vi "Actor Core.vi"(8 "error in":errorcluster, 11 "Recipe Window in":refnum<class "Recipe Window.lvclass">) -> (0 "error out":errorcluster, 3 "Actor out":refnum<class "Actor.lvclass">)   [LabVIEW 2021, in "Recipe.lvlib" / "Recipe Window.lvclass"]
doc: "The user interface for this panel.\n\n----\nPlease see the following web address for additional documentation and tutorial information:\nhttp://www.mooregoodideas.com/mgi-panel-manager/\n\nAuthor: Derek Trepanier\n\nCopyright (c) 2018, Moore Good Ideas, Inc.\n\nAll rights reserved.\n\nRedistribution and use in source and binary forms, with or without modification, are permitted provided that the following conditions are met:\n\n * Redistributions of source code must retain the above copyright notice, this list of conditions and the following disclaimer.\n * Redistributions in binary form must reproduce the above copyright notice, this list of conditions and the following disclaimer in the documentation and/or other materials provided with the distribution.\n * Neither the name of Moore Good Ideas, Inc. nor the names of its contributors may be used to endorse or promote products derived from this software without specific prior written permission.\n\nTHIS SOFTWARE IS PROVIDED BY THE COPYRIGHT HOLDERS AND CONTRIBUTORS \"AS IS\" AND ANY EXPRESS OR IMPLIED WARRANTIES, INCLUDING, BUT NOT LIMITED TO, THE IMPLIED WARRANTIES OF MERCHANTABILITY AND FITNESS FOR A PARTICULAR PURPOSE ARE DISCLAIMED. IN NO EVENT SHALL THE COPYRIGHT OWNER OR CONTRIBUTORS BE LIABLE FOR ANY DIRECT, INDIRECT, INCIDENTAL, SPECIAL, EXEMPLARY, OR CONSEQUENTIAL DAMAGES (INCLUDING, BUT NOT LIMITED TO, PROCUREMENT OF SUBSTITUTE GOODS OR SERVICES; LOSS OF USE, DATA, OR PROFITS; OR BUSINESS INTERRUPTION) HOWEVER CAUSED AND ON ANY THEORY OF LIABILITY, WHETHER IN CONTRACT, STRICT LIABILITY, OR TORT (INCLUDING NEGLIGENCE OR OTHERWISE) ARISING IN ANY WAY OUT OF THE USE OF THIS SOFTWARE, EVEN IF ADVISED OF THE POSSIBILITY OF SUCH DAMAGE."
uses:
  Recipe Window.lvclass
  <vilib>/ActorFramework/Stop Msg/Stop Msg.lvclass
  <vilib>/MGI/Panel Manager/Panel Actor/Panel Actor/Panel Actor.lvclass
  Recipe Window Messages/Recipe Label Changed-Event Msg/Recipe Label Changed-Event Msg.lvclass
  Recipe Window Messages/Body Pane Resized-Event Msg/Body Pane Resized-Event Msg.lvclass
  C:/Program Files (x86)/National Instruments/LabVIEW 2021/vi.lib/MGI/Panel Manager/Panel Actor/Panel Actor/Panel Actor.lvclass
  C:/Program Files (x86)/National Instruments/LabVIEW 2021/vi.lib/MGI/Monitored Actor/Monitored Actor/Monitored Actor/Monitored Actor.lvclass
  C:/Program Files (x86)/National Instruments/LabVIEW 2021/vi.lib/ActorFramework/Actor/Actor.lvclass
  C:/Users/Thomas/Documents/Projects/Recipe/Actors/Recipe Window/Recipe Window.lvclass
  <vilib>/ActorFramework/Actor/Actor.lvclass
  Typedefs/Recipe Line--cluster.ctl
panel:
  in  "Recipe Label":string
  in  "String":string
  in  "Recipe Line":T1
  in  "New Line":bool
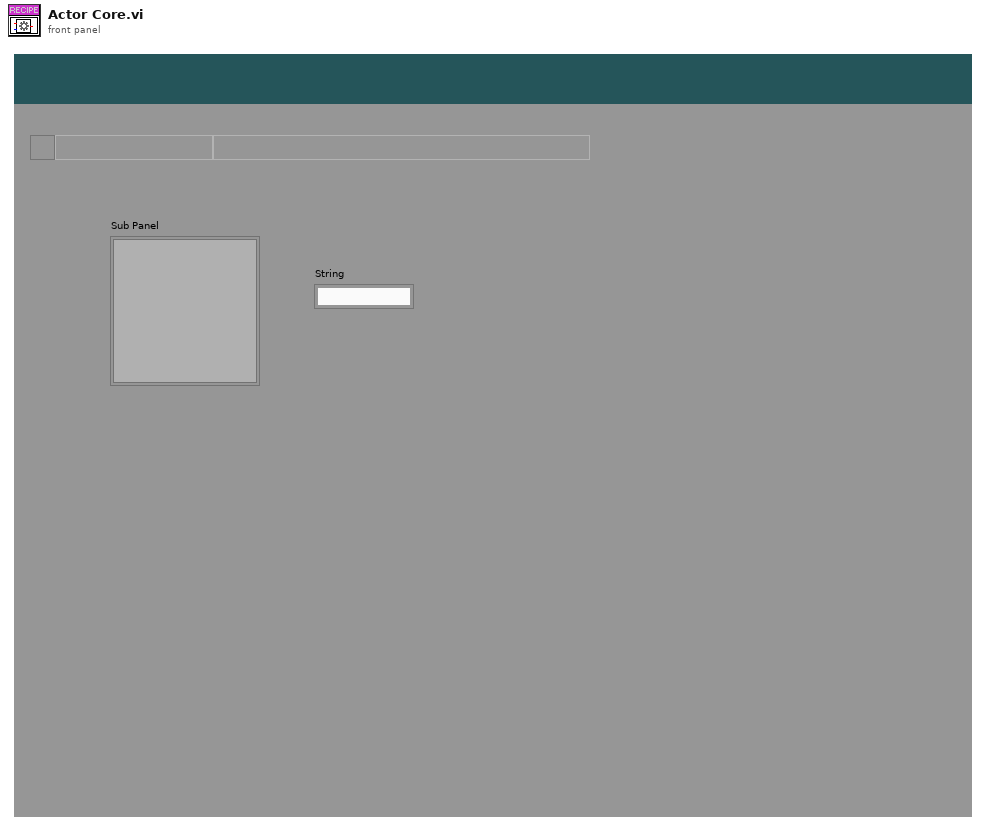
[diagram p1: front panel]
types:
  T1 = typedef "Recipe.lvlib/Recipe Window.lvclass/Recipe Line--cluster.ctl" = cluster{"Checkbox 2":bool, "Title":string, "Comment":string, "Drag":bool}
  T2 = cluster{"Pnl Actor":refnum<event-registration>, "Pnl Events":refnum<event-registration>}
  T3 = typedef "LVRectTypeDef.ctl" = cluster{"Left":i16, "Top":i16, "Right":i16, "Bottom":i16}
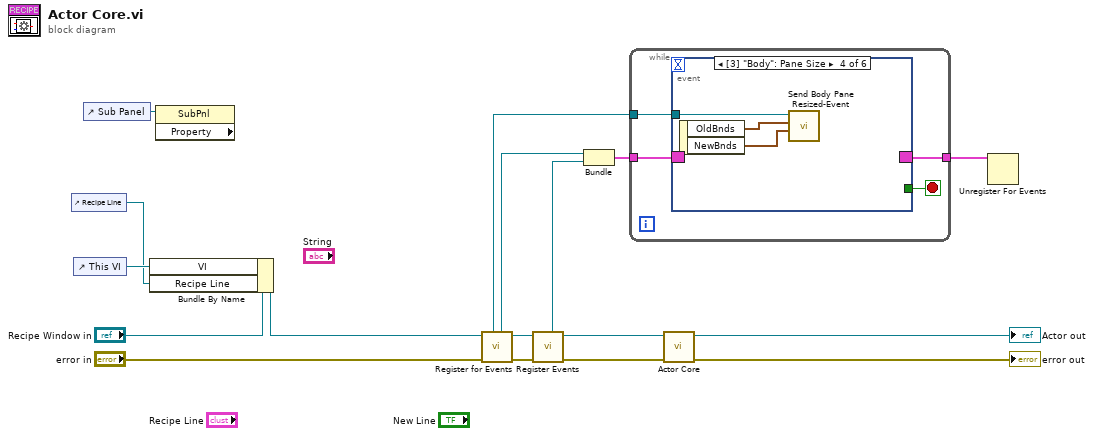
[diagram p0: block diagram]
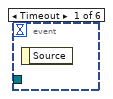
[diagram p2: hidden frame]
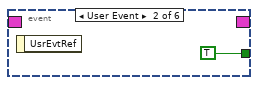
[diagram p3: hidden frame]
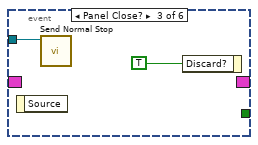
[diagram p4: hidden frame]
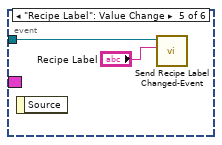
[diagram p5: hidden frame]
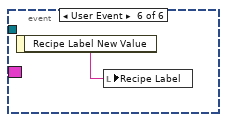
[diagram p6: hidden frame]
diagram:
  n1 = control-ref of="Recipe Line"() -> (w2:refnum<vi>)
  n2 = control-ref of="This VI"() -> (w10:refnum<vi>)
  n3 = control-ref of="Sub Panel"() -> (w1:refnum<vi>)
  n4 = Bundle By Name(cluster="Recipe Window in", "VI"=w10, "Recipe Line"=w2) -> (w9:refnum<class "Recipe Window.lvclass">)
  n5 = property class="SubPnl" props=[](reference=w1) -> ()  [unwired: 1 in, 3 out]
  n6 = call <vilib>:"Register for Events.vi"("Error In"="error in", "Panel Actor in"=w9) -> ("Error Out"=w14:errorcluster, "Panel Actor out"=w5:refnum<class "Recipe Window.lvclass">, "Pnl Actor"=w7:refnum<event-registration>, "Self Enqueuer"=w13:refnum<class "Message Enqueuer.lvclass">)  [unwired: 6 in]
  n7 = call "Register Events.vi"("error in (no error)"=w14, "Recipe Window in"=w5) -> ("error out"=w6:errorcluster, "Recipe Window out"=w4:refnum<class "Recipe Window.lvclass">, "Pnl Events"=w3:refnum<event-registration>)  [unwired: 7 in]
  n8 = Bundle("Pnl Actor"=w7, "Pnl Events"=w3) -> (w8:T2)  [unwired: 1 in]
  n9 = while {
    tunnel: w8 -> [w21]
    tunnel: w13 -> [w20]
    tunnel: [w18] -> w15
    stop <- w19 stop-if-true
    n10 = event shown="[3] \"Body\": Pane Size" {
      selector: w21 -> [_ _ _ _ _ _]
      dyn-events: [_ _ _ _ _ _] -> w18
      timeout: _ -> [_ _ _ _ _ _]
      tunnel: w20 -> [_ _ w24 w27 w29 _]
      tunnel: [_ TRUE _ _ _ _] -> w19
      event Timeout {
        n11 = event-data() -> ()  [unwired: 1 in, 1 out]
      }
      event User Event {
        n12 = event-data() -> ()  [unwired: 1 in, 1 out]
      }
      event Panel Close? {
        n13 = event-data() -> ()  [unwired: 1 in, 1 out]
        n14 = call <vilib>:"Send Normal Stop.vi"("Message Enqueuer"=w24) -> ()  [unwired: 10 in, 1 out]
        n15 = event-data("Discard?"=TRUE) -> ()  [unwired: 1 in, 1 out]
      }
      event Pane Size {
        n16 = event-data() -> ("OldBnds"=w26:T3, "NewBnds"=w25:T3)  [unwired: 1 in]
        n17 = call "Send Body Pane Resized-Event.vi"("NewBnds"=w25, "OldBnds"=w26, "Message Enqueuer"=w27) -> ()  [unwired: 7 in, 2 out]
      }
      event "Recipe Label": Value Change {
        n18 = event-data() -> ()  [unwired: 1 in, 1 out]
        n19 = call "Send Recipe Label Changed-Event.vi"("New Label"="Recipe Label", "Message Enqueuer"=w29) -> ()  [unwired: 8 in, 2 out]
      }
      event User Event {
        n20 = event-data() -> ("Recipe Label New Value"=w30:string)  [unwired: 1 in]
        n21 = local write "Recipe Label"(w30) -> ()
      }
    }
  }
  n22 = call-parent "Actor Core.vi"("error in"=w6, "Panel Actor in"=w4) -> ("error out"=→"error out":errorcluster, "Actor out"=→"Actor out":refnum<class "Actor.lvclass">)  [unwired: 8 in]
  n23 = Unregister For Events(event registration refnum=w15) -> ()  [unwired: 1 in, 1 out]
